vi "SPC_get_time_from_start.vi"(8 "Error In":errorcluster, 10 "Module No":i16 min=0 max=7 step=1, 11 "DLL Path":path) -> (0 "Error Out":errorcluster, 2 "Module No":i16 min=0 max=7 step=1, 3 "DLL Path":path, 4 "Time Value":sgl format="%.2f")   [LabVIEW 2023]
doc: "The procedure reads the SPC repeat timer and calculates the time from the start of the \nmeasurement for the SPC module ‘mod_no’. It should be called during the measurement, \nbecause the timer starts to run after (re)starting the measurement.\nFor collection times longer than 80 seconds be sure that SPC_test_state is called in the loop during the measurement before the SPC_get_time_from_start call. SPC_test_state updates software counter which is needed for times longer than 80 sec.\nThe procedure can be used to test the progress of the measurement or to the start next measurement step in a multi-step measurements (such as f(t,T) in the standard software).\nWhen the sequencer is running the repeat timer is not available. In this case SPC_get_time_from_start uses a software timer to measure the time from the start of the measurement\n\ninfo@becker-hickl.com"
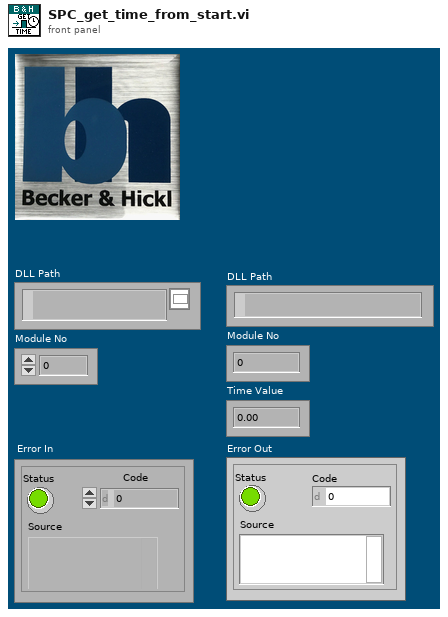
[diagram p1: front panel]
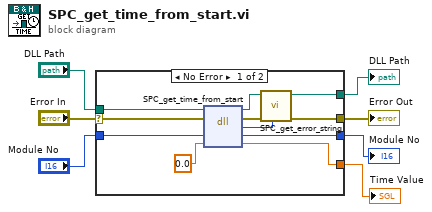
[diagram p0: block diagram]
diagram:
  n1 = case shown="No Error" "Error In" {
    selector: "Error In" -> [w17 w20]
    tunnel: "DLL Path" -> [w18 w21]
    tunnel: [w15 w20] -> w5
    tunnel: [w12 w21] -> w4
    tunnel: "Module No" -> [w11 w19]
    tunnel: [w10 w19] -> w2
    tunnel: [w8 _] -> w1
    frame No Error {
      n2 = dll-call lib="D:/spcm/lib/lab_view/lv10.0/spcm32.dll" fn="SPC_get_time_from_start"(path in=w18, error in=w17, "mod_no"=w11, "time"=sgl 0.0 ("Last Time Value")) -> (path out=w13:path, error out=w16:errorcluster, "return type"=w14:i16, "mod_no"=w10:i16, "time"=w8:sgl)  [unwired: 1 in]
      n3 = call "SPC_get_error_string.vi"("ErrorID"=w14, "Error In"=w16, "DLL Path"=w13) -> ("Error Out"=w15:errorcluster, "DLL Path"=w12:path)  [unwired: 6 in, 1 out]
    }
    frame Error {
    }
  }
  "Error Out" <- w5
  "DLL Path" <- w4
  "Module No" <- w2
  "Time Value" <- w1
